vi "Lab1_tutorial.vi"() -> ()   [LabVIEW 2010]
uses:
  <vilib>/Platform/TimedLoop/XDataNode/XDataNode.xnode
  <vilib>/Platform/TimedLoop/XDataNode/timing_clust.ctl
  <vilib>/Platform/TimedLoop/XDataNode/nitl_modes.ctl
  <vilib>/Platform/TimedLoop/XDataNode/wakeup.ctl
  <vilib>/Platform/TimedLoop/XDataNode/XDNodeRunTimeDep.lvlib
panel:
  out "Waveform Chart":dynamicdata(graph)
  in  "Phase (Degrees)":dbl
  in  "DC Offset":dbl
  in  "Amplitude":dbl
  in  "Frequency (Hz)":dbl
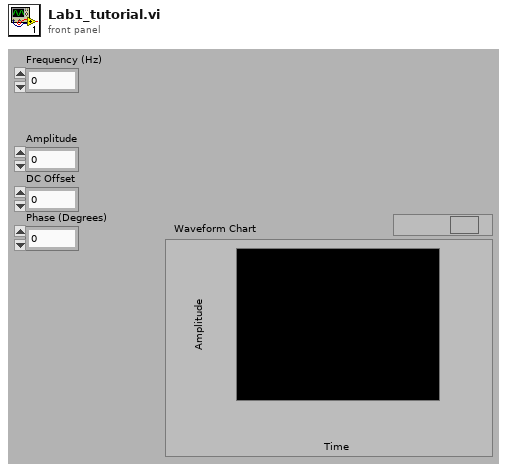
[diagram p1: front panel]
types:
  T1 = typedef "XDNodeRunTimeDep.lvlib/timing_clust.ctl" = cluster{"Expected End [f-1]":u64, "Actual End [f-1]":u64, "Finished Late? [f-1]":bool, "Expected End [i-1]":u64, "Actual End [i-1]":u64, "Finished Late? [i-1]":bool, "Expected Start [i]":u64, "Actual Start [i]":u64, "Expected Start [f]":u64, "Actual Start [f]":u64, "Source Name":string, "Structure Name":string, "Period":i64, "Deadline":i64, "Offset":i64, "Start":i64, "Priority":i32, "Timeout":i32, "Mode":T2, "Wakeup Reason":T3, "Error":errorcluster, "Source Type":string, "Secondary Source Type":string, "Global End Time":u64, "Global Start Time":u64, "Frame Duration":u64, "Iteration Duration":u64, "Assigned CPU":i32, "I/O Scan Engine Mode":u32}
  T2 = typedef "XDNodeRunTimeDep.lvlib/nitl_modes.ctl" = enum32{"No Change", "Process missed periods, maintain original phase", "Discard missed periods, maintain original phase", "Process missed periods, ignore original phase", "Discard missed periods, ignore original phase"}
  T3 = typedef "XDNodeRunTimeDep.lvlib/wakeup.ctl" = enum32{"Normal", "Aborted", "Asynchronous wakeup", "Timing source error", "Timed loop error", "Timeout"}
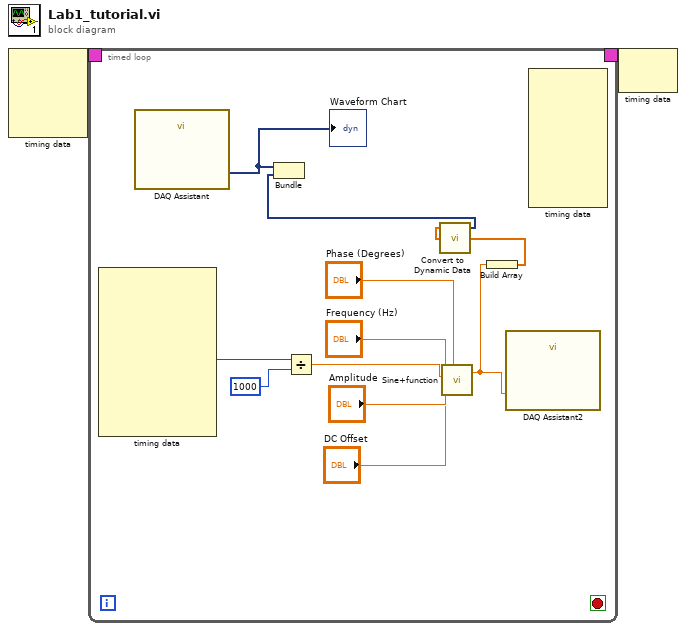
[diagram p0: block diagram]
diagram:
  n1 = node-c288() -> (w2:T1)  [unwired: 4 in]
  n2 = timed-loop {
    timing: w2 -> [_]
    timing-out: [_] -> w1
    stop <- _ stop-if-true
    n3 = node-c288() -> (w9:i64)  [unwired: 1 in, 9 out]
    n4 = call "DAQ Assistant"() -> ("data"=w3:dynamicdata)  [unwired: 17 in, 2 out]
    "Waveform Chart" <- w3
    n5 = Divide(x=w9, y=1000) -> (x/y=w7:dbl)
    n6 = call "Sine+function.vi"("Frequency (Hz)"="Frequency (Hz)", "Time (Sec)"=w7, "Amplitude"="Amplitude", "DC Offset"="DC Offset", "Phase (Degrees)"="Phase (Degrees)") -> ("A*sin(2*pi*f*t+phi)+B"=w6:dbl)  [unwired: 1 in]
    n7 = Build Array(w6) -> (w5:dbl[])
    n8 = call "Convert to Dynamic Data"("Array"=w5) -> ("Dynamic Data Type"=w4:dynamicdata)  [unwired: 3 in]
    n9 = Bundle("data"=w3, "Dynamic Data Type"=w4) -> ()  [unwired: 1 in, 1 out]
    n10 = call "DAQ Assistant2"("data"=w6) -> ()  [unwired: 17 in, 2 out]
    n11 = node-c288() -> ()  [unwired: 8 in, 1 out]
  }
  n12 = node-c288(w1) -> ()  [unwired: 1 out]
